vi "Read Measurements.vi"   [LabVIEW 2014, in "Associated Power Technologies 8500 Series.lvlib"]
doc: "Reads the test data individually from the instrument during the test progress."
uses:
  <instrlib>/Associated Power Technologies 8500 Series/Associated Power Technologies 8500 Series.lvlib
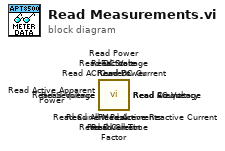
[diagram p0: block diagram]
diagram:
  n1 = call <instrlib>:"Read All Measurements.vi"() -> ()  [unwired: 13 in, 3 out]
  n2 = call <instrlib>:"Read DC Current.vi"() -> ()  [unwired: 13 in, 3 out]
  n3 = call <instrlib>:"Read Sequence.vi"() -> ()  [unwired: 13 in, 3 out]
  n4 = call <instrlib>:"Read Count.vi"() -> ()  [unwired: 13 in, 3 out]
  n5 = call <instrlib>:"Read Dwell Time.vi"() -> ()  [unwired: 13 in, 3 out]
  n6 = call <instrlib>:"Read State.vi"() -> ()  [unwired: 13 in, 3 out]
  n7 = call <instrlib>:"Read AC Current.vi"() -> ()  [unwired: 13 in, 3 out]
  n8 = call <instrlib>:"Read DC Voltage.vi"() -> ()  [unwired: 13 in, 3 out]
  n9 = call <instrlib>:"Read AC Voltage.vi"() -> ()  [unwired: 13 in, 3 out]
  n10 = call <instrlib>:"Read Active Apparent Power.vi"() -> ()  [unwired: 13 in, 3 out]
  n11 = call <instrlib>:"Read Crest Factor.vi"() -> ()  [unwired: 13 in, 3 out]
  n12 = call <instrlib>:"Read Active Reactive Current.vi"() -> ()  [unwired: 13 in, 3 out]
  n13 = call <instrlib>:"Read Current Peak.vi"() -> ()  [unwired: 13 in, 3 out]
  n14 = call <instrlib>:"Read Power Factor.vi"() -> ()  [unwired: 13 in, 3 out]
  n15 = call <instrlib>:"Read Power.vi"() -> ()  [unwired: 13 in, 3 out]
  n16 = call <instrlib>:"Read Current.vi"() -> ()  [unwired: 13 in, 3 out]
  n17 = call <instrlib>:"Read Frequency.vi"() -> ()  [unwired: 13 in, 3 out]
  n18 = call <instrlib>:"Read Voltage.vi"() -> ()  [unwired: 13 in, 3 out]
